vi "Set Customer Work Dispatchers.vi"(8 "error in (no error)":errorcluster, 10 "Customer":refnum<class "Customer.lvclass">, 11 "Coffee Shop In":refnum<class "Coffee Shop.lvclass">) -> (0 "error out":errorcluster, 3 "Coffee Shop Out":refnum<class "Coffee Shop.lvclass">)   [LabVIEW 2020, in "Coffee Shop.lvclass"]
uses:
  Coffee Shop.lvclass
  C:/Program Files (x86)/National Instruments/LabVIEW 2020/vi.lib/Astemes/Triarc Framework/Process/Process.lvclass
  People/Customers/Customer/Customer.lvclass
  <vilib>/Astemes/Triarc Framework/Process/Process.lvclass/Process.ctl
  <vilib>/Astemes/Triarc Framework/Process/Private/SubVIs/Handle Debug Data.vi
  <vilib>/Astemes/Triarc Framework/Logging/Log Debug.vi
  <vilib>/AdvancedString/1D String Array to Delimited String.vi
  <vilib>/Utility/High Resolution Relative Seconds.vi
  <vilib>/Astemes/Triarc Framework/Process/Public/Read Name.vi
  <vilib>/Astemes/Triarc Framework/Callback/Callback.lvclass
  <vilib>/Astemes/Triarc Framework/Process/Process.lvclass
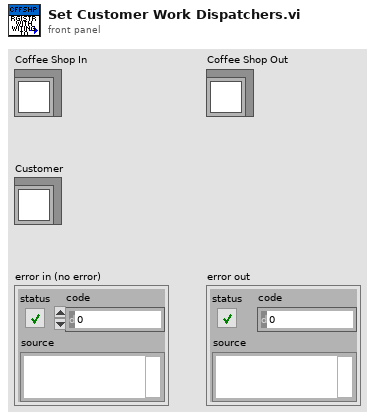
[diagram p1: front panel]
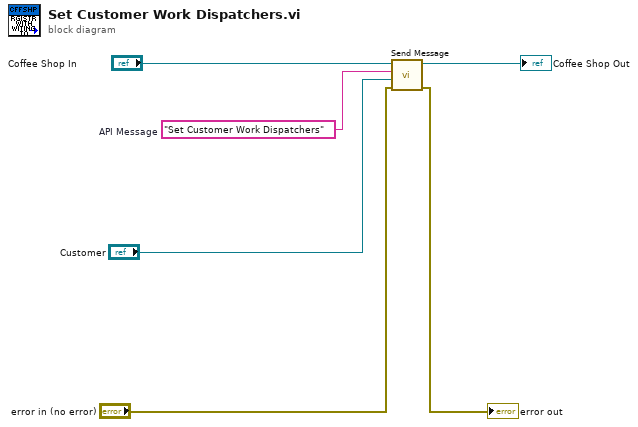
[diagram p0: block diagram]
diagram:
  w3 = "Set Customer Work Dispatchers"  # API Message
  n1 = call <vilib>:"Send Message.vi"("error in (no error)"="error in (no error)", "Message Data"="Customer", "Message"=w3, "Process In"="Coffee Shop In") -> ("error out"=→"error out":errorcluster, "Process Out"=→"Coffee Shop Out":refnum<class "Coffee Shop.lvclass">)  [unwired: 6 in]
